vi "SaveImage.vi"(8 "error in (no error)":errorcluster, 9 "IndexOfImages":i32, 10 "Image Dst In":T1, 11 "FileOperation in":refnum<class "FileOperation.lvclass">) -> (0 "error out":errorcluster, 3 "FileOperation out":refnum<class "FileOperation.lvclass">)   [LabVIEW 2015, in "FileOperation.lvclass"]
uses:
  FileOperation.lvclass
  <vilib>/vision/Image Controls.llb/IMAQ Image.ctl
  FileOperation.lvclass/FileOperation.ctl
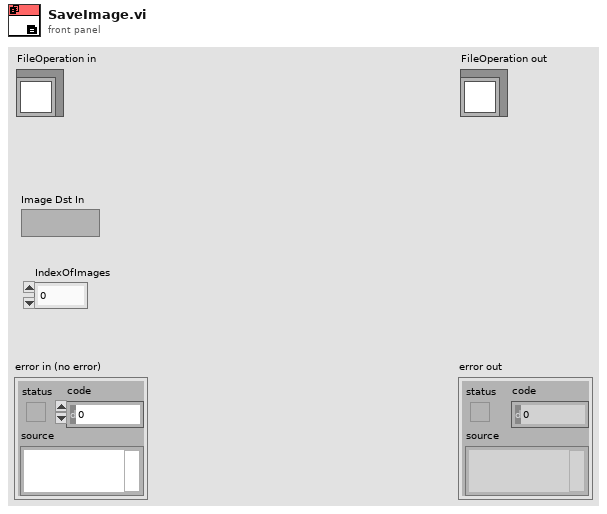
[diagram p1: front panel]
types:
  T1 = typedef "IMAQ Image.ctl" = refnum<image>
  T2 = enum16{"open", "replace", "create", "open or create", "replace or create", "replace or create with confirmation"}
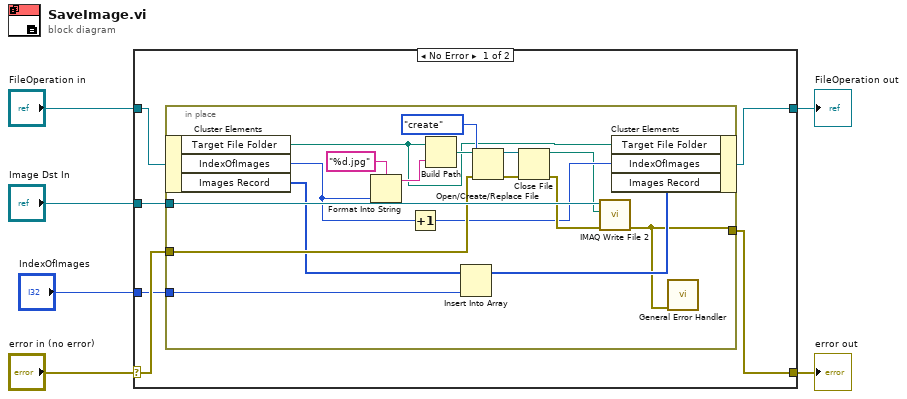
[diagram p0: block diagram]
diagram:
  n1 = case shown="No Error" "error in (no error)" {
    selector: "error in (no error)" -> [w10 w31]
    tunnel: [w8 w31] -> w5
    tunnel: [w9 w30] -> w3
    tunnel: "FileOperation in" -> [w11 w30]
    tunnel: "Image Dst In" -> [w12 _]
    tunnel: "IndexOfImages" -> [w7 _]
    frame No Error {
      n2 = in-place {
        in-place-border: w12 -> [w29]
        in-place-border: w10 -> [w24]
        in-place-border: [w17] -> w8
        in-place-border: w7 -> [w19]
        n3 = in-place-cluster #1(w11) -> ("Target File Folder"=w14:path, "IndexOfImages"=w16:i32, "Images Record"=w20:i32[])
        n4 = Format Into String(format string="%d.jpg", w16) -> (resulting string=w27:string)  [unwired: 2 in, 1 out]
        n5 = Increment(x=w16) -> (x+1=w15:i32)
        n6 = Build Path(base path=w14, name or relative path=w27) -> (appended path=w26:path)
        n7 = Insert Into Array(array=w20, new element=w19) -> (w18:i32[])  [unwired: 1 in]
        n8 = Open/Create/Replace File(file path (use dialog)=w26, error in=w24, operation (0:open)=T2."create") -> (refnum out=w22:refnum<file>, error out=w23:errorcluster)  [unwired: 3 in, 1 out]
        n9 = Close File(refnum=w22, error in=w23) -> (path=w13:path, error out=w21:errorcluster)
        n10 = call-poly "IMAQ Write File 2"("error in (no error)"=w21, "File Path"=w13, "Image"=w29) -> ("error out"=w17:errorcluster)  [unwired: 7 in, 1 out]
        n11 = in-place-cluster #1("Target File Folder"=w14, "IndexOfImages"=w15, "Images Record"=w18) -> (w9:refnum<class "FileOperation.lvclass">)
        n12 = call <vilib>:"General Error Handler.vi"("error in (no error)"=w17) -> ()  [unwired: 10 in, 5 out]
      }
    }
    frame Error {
    }
  }
  "error out" <- w5
  "FileOperation out" <- w3
